vi "Check File Existence.vi"(8 "error in (no error)":errorcluster, 11 "Config_Read_SPI.lvclass":refnum<class "Config_Read_SPI.lvclass">) -> (0 "error out":errorcluster, 3 "Config_Read_SPI.lvclass out":refnum<class "Config_Read_SPI.lvclass">)   [LabVIEW 2018, in "Config_Read_SPI.lvclass"]
uses:
  Config_Read_SPI.lvclass
  Config_Read_SPI.lvclass/Config_Read_SPI.ctl
  Classes/Config_Read/Config_Read_BML.lvclass
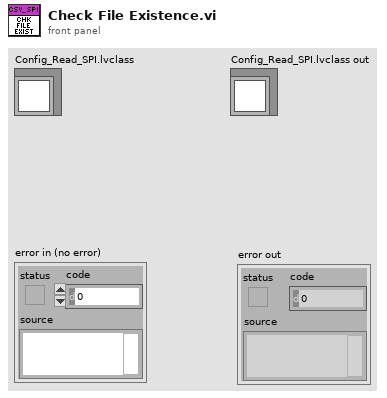
[diagram p1: front panel]
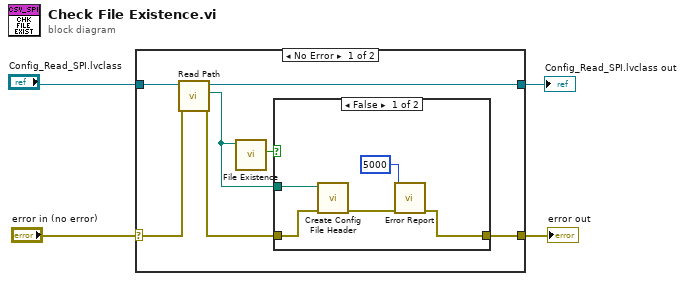
[diagram p0: block diagram]
diagram:
  n1 = case shown="No Error" "error in (no error)" {
    selector: "error in (no error)" -> [w6 w18]
    tunnel: [w11 w18] -> w3
    tunnel: [w8 w19] -> w1
    tunnel: "Config_Read_SPI.lvclass" -> [w9 w19]
    frame No Error {
      n2 = call "Read Path.vi"("error in (no error)"=w6, "Config_Read_SPI in"=w9) -> ("error out"=w5:errorcluster, "Path"=w7:path, "Config_Read_SPI out"=w8:refnum<class "Config_Read_SPI.lvclass">)  [unwired: 7 in]
      n3 = call "File Existence"("file path"=w7) -> ("exists"=w10:bool)  [unwired: 9 in, 1 out]
      n4 = case shown="False" w10 {
        tunnel: w7 -> [w14 _]
        tunnel: [w15 w17] -> w11
        tunnel: w5 -> [w13 w17]
        frame False {
          n5 = call "Create Config File Header.vi"("error in (no error)"=w13, "file path"=w14) -> ("error out"=w12:errorcluster)  [unwired: 8 in, 1 out]
          n6 = call "Error Report.vi"("error in (no error)"=w12, "Error Code"=i16 5000) -> ("error out"=w15:errorcluster)  [unwired: 9 in]
        }
        frame True {
        }
      }
    }
    frame Error {
    }
  }
  "error out" <- w3
  "Config_Read_SPI.lvclass out" <- w1
